vi "Difference Matrix Generator.vi"(11 "Graph Matrix":T1) -> (0 "Minimum distances between vertices":i32[][](array[numeric]), 1 "Difference Between Labels Matrix":i32[][](array[numeric]), 2 "Diameter":i32, 3 "Disconnected!":bool=TRUE)   [LabVIEW 2016]
uses:
  <vilib>/Analysis/Matrix/Datatypes/RealMatrix.ctl
  <vilib>/Analysis/Matrix/Numeric/Power Of X/Power Of X - RM,I.vi
  <vilib>/Analysis/Matrix/NI_Matrix.lvlib
panel:
  # "The main diagonal isn't useful here"
  # "Must be a square matrix"
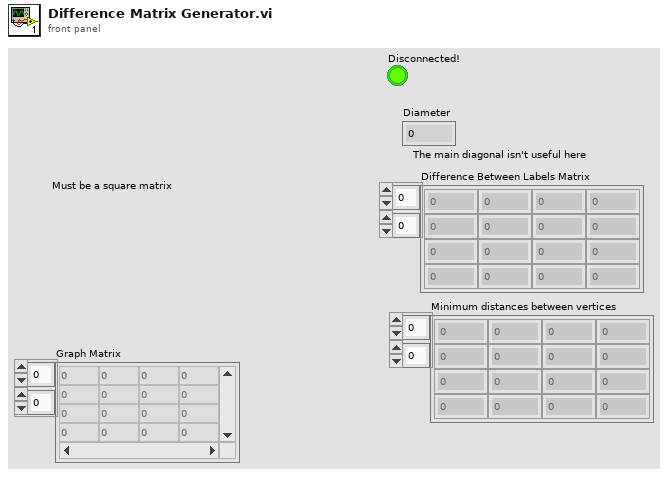
[diagram p1: front panel]
types:
  T1 = typedef "NI_Matrix.lvlib/RealMatrix.ctl" = dbl[][]
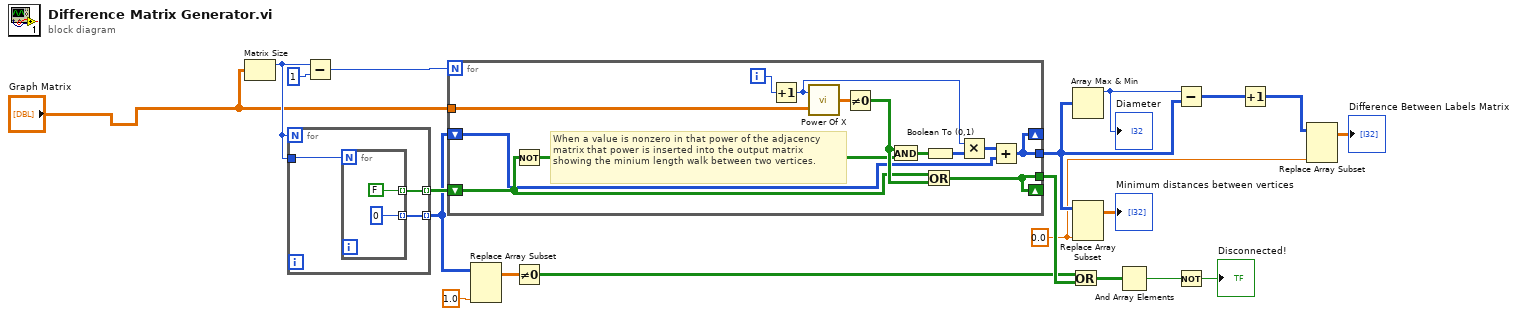
[diagram p0: block diagram]
diagram:
  w2 = 0.0 ("new diagonal/fill element")
  n1 = Matrix Size(0:"Graph Matrix") -> (1:w14:i32)  [unwired: 1 out]
  n2 = for {
    N: w14 -> [_]
    tunnel: w14 -> [w23]
    tunnel: [w22] -> w12 mode=indexing
    tunnel: [w21] -> w11 mode=indexing
    n3 = for {
      N: w23 -> [_]
      tunnel: [FALSE] -> w22 mode=indexing
      tunnel: [0] -> w21 mode=indexing
    }
  }
  n4 = Subtract(x=w14, y=1) -> (x-y=w19:i32)
  n5 = for {
    N: w19 -> [_]
    tunnel: "Graph Matrix" -> [w38]
    shift-right: [w27] -> _
    shift-left: w12 -> [w35]
    shift-right: [w28] -> _
    shift-left: w11 -> [w29]
    tunnel: [w28] -> w6
    tunnel: [w27] -> w18
    i -> [w31]
    # "When a value is nonzero in that power of the adjacency matrix that power is inserted into the output matrix showing the minium length walk between two vertices."
    n6 = Not(x=w35) -> (.not. x?=w34:bool[][])
    n7 = Increment(x=w31) -> (x+1=w26:i32)
    n8 = call-poly <vilib>:"Power Of X.vi"("Real Matrix A"=w38, "Power n"=w26) -> ("A^n"=w37:T1)
    n9 = Not Equal To 0?(x=w37) -> (x != 0?=w36:bool[][])
    n10 = And(x=w36, y=w34) -> (x .and. y?=w33:bool[][])
    n11 = Or(x=w35, y=w36) -> (x .or. y?=w27:bool[][])
    n12 = Boolean To (0,1)(Boolean=w33) -> (0, 1=w32:i16[][])
    n13 = Multiply(x=w26, y=w32) -> (x*y=w30:i32[][])
    n14 = Add(x=w30, y=w29) -> (x+y=w28:i32[][])
  }
  n15 = Replace Array Subset(array=w11, new element=1.0 ("new diagonal/fill element")) -> (w9:T1)  [unwired: 2 in]
  n16 = Not Equal To 0?(x=w9) -> (x != 0?=w7:bool[][])
  n17 = Or(x=w7, y=w18) -> (x .or. y?=w8:bool[][])
  n18 = Array Max & Min(array=w6) -> (max value=w16:i32)  [unwired: 3 out]
  "Diameter" <- w16
  n19 = Replace Array Subset(array=w6, new element=w2) -> (→"Minimum distances between vertices":T1)  [unwired: 2 in]
  n20 = And Array Elements(Boolean array=w8) -> (logical AND=w17:bool)
  n21 = Subtract(x=w16, y=w6) -> (x-y=w15:i32[][])
  n22 = Not(x=w17) -> (.not. x?=→"Disconnected!":bool)
  n23 = Increment(x=w15) -> (x+1=w4:i32[][])
  n24 = Replace Array Subset(array=w4, new element=w2) -> (→"Difference Between Labels Matrix":T1)  [unwired: 2 in]
